vi "灯值调整对话框.vi"() -> ()   [LabVIEW 2016, in "斯坦道CODcr.lvlib"]
uses:
  <vilib>/Plasmionique/MB Master/MB_Master/MB_Master.lvclass
panel:
  out "工作状态:":string
  in  "纯水填充":bool
  out "660 阻值":u16 caption="660 阻值："
  out "520 阻值":u16 caption="520 阻值："
  out "365 阻值":u16 caption="365 阻值："
  in  "停止":bool
  in  "校准":bool
  out "校准状态":u16(ring) caption="调灯状态：" items=["空闲", "校准中"]
  out "当前阻值":u16 caption="当前阻值："
  out "当前光强":u16 caption="当前光强："
  in  "目标光强":u16=3300 caption="目标光强："
  in  "灯类型":enum32{"365", "520", "660"}(radio)=enum."660" caption="灯类型："
  # "365：海水氨氮\n520：海水氨氮、氨氮总磷（氨氮光源）\n660：总磷、氨氮"
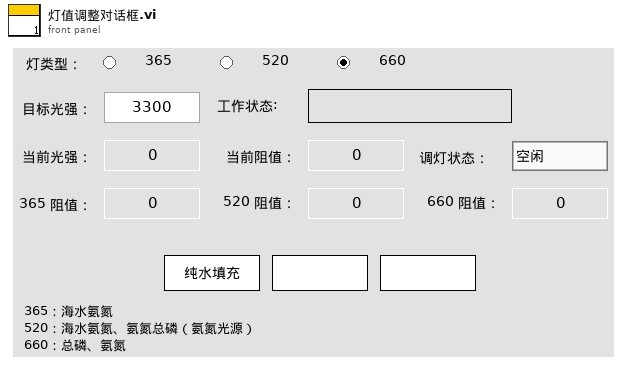
[diagram p1: front panel]
types:
  T1 = enum8{"Enabled", "Disabled", "Disabled and Grayed Out"}
  T2 = cluster{"系统时间":timestamp, "工作状态":u16, "测量模式":enum16{"待机", "连续模式", "周期模式", "定点模式", "受控模式", "手动模式"}, "告警代码":u16, "故障代码":u16, "日志代码":u16, "软件版本":u16, "F0":sgl, "F1":sgl, "F2":sgl, "F3":sgl, "T":sgl, "H":sgl, "id":u16, "flowid":u16, "量程":u16, "总磷控温温度1":sgl, "营养盐控温温度2":sgl, "ADC":sgl}
  T3 = cluster{"360 阻值":u16, "520 阻值":u16, "660 阻值":u16}
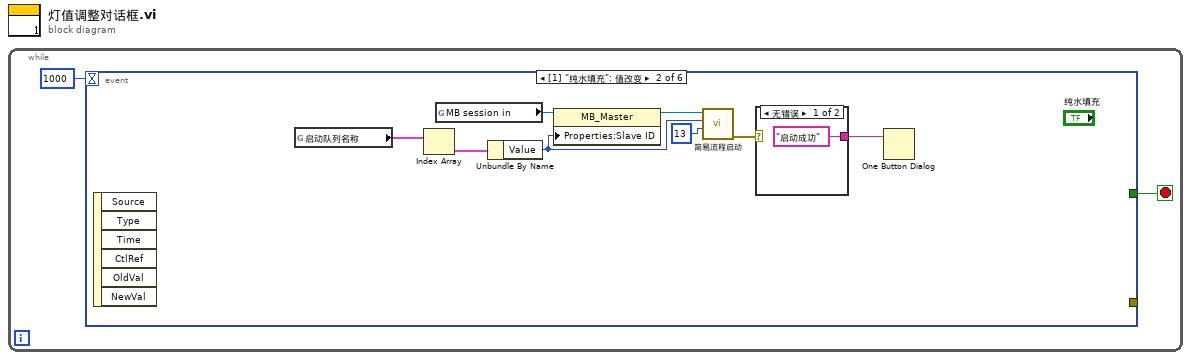
[diagram p0: block diagram]
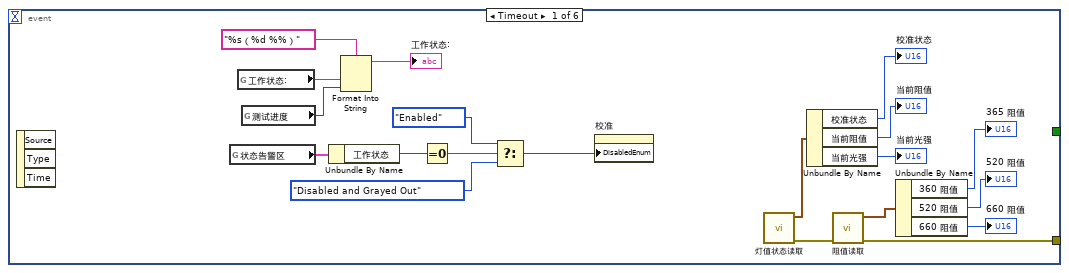
[diagram p2: hidden frame]
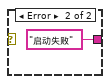
[diagram p3: hidden frame]
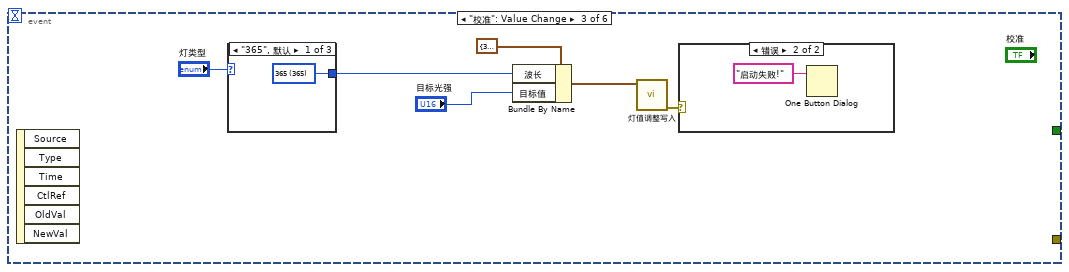
[diagram p4: hidden frame]
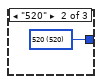
[diagram p6: hidden frame]
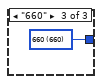
[diagram p7: hidden frame]
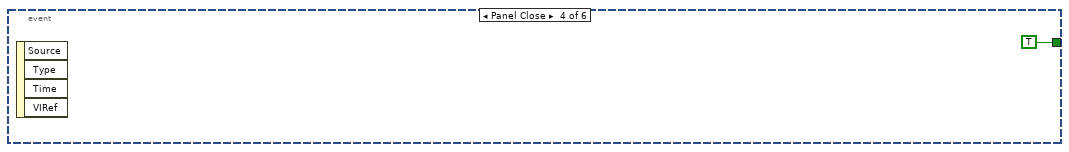
[diagram p8: hidden frame]
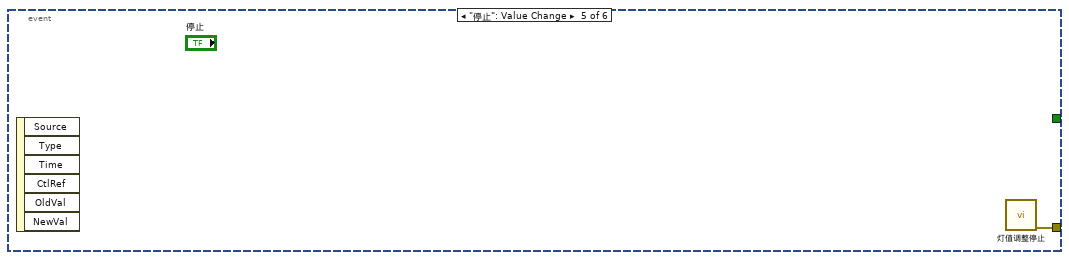
[diagram p9: hidden frame]
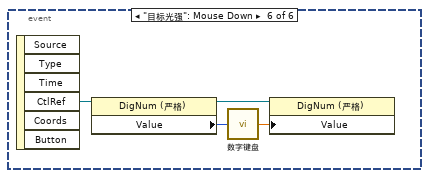
[diagram p10: hidden frame]
diagram:
  n1 = while {
    stop <- w2 stop-if-true
    n2 = event shown="[1] \"纯水填充\": 值改变" {
      selector: _ -> [_ _ _ _ _ _]
      dyn-events: _ -> [_ _ _ _ _ _]
      timeout: 1000 -> [_ _ _ _ _ _]
      tunnel: [_ _ _ TRUE _ _] -> w2
      tunnel: [w13 _ _ _ w44 _] -> _
      event Timeout {
        n3 = event-data() -> ()  [unwired: 1 in, 3 out]
        n4 = global read "VAR总磷总氮全局变量.vi" "状态告警区"() -> (w12:T2)
        n5 = global read "VAR总磷总氮全局变量.vi" "工作状态:"() -> (w5:string)
        n6 = global read "VAR总磷总氮全局变量.vi" "测试进度"() -> (w4:u8)
        n7 = Unbundle By Name(w12) -> ("工作状态"=w11:u16)
        n8 = Format Into String(format string="%s（%d %%）" ("格式字符串"), w5, w4) -> (resulting string=→"工作状态:":string)  [unwired: 2 in, 1 out]
        n9 = Equal To 0?(x=w11) -> (x = 0?=w10:bool)
        n10 = Select(t=T1."Enabled" ("禁用"), s=w10, f=T1."Disabled and Grayed Out") -> (s? t:f=w8:T1)
        n11 = property on="校准" class="Bool"("DisabledEnum"=w8) -> ()  [unwired: 2 in, 2 out]
        n12 = call "灯值状态读取.vi"() -> ("error out"=w22:errorcluster, "状态值"=w21:cluster{"校准状态":u16, "当前阻值":u16, "当前光强":u16})  [unwired: 10 in]
        n13 = Unbundle By Name(w21) -> ("校准状态"=→"校准状态":u16, "当前阻值"=→"当前阻值":u16, "当前光强"=→"当前光强":u16)
        n14 = call "阻值读取.vi"("error in (no error)"=w22) -> ("error out"=w13:errorcluster, "状态值"=w17:T3)  [unwired: 9 in]
        n15 = Unbundle By Name(w17) -> ("360 阻值"=→"365 阻值":u16, "520 阻值"=→"520 阻值":u16, "660 阻值"=→"660 阻值":u16)
      }
      event "纯水填充": Value Change {
        n16 = event-data() -> ()  [unwired: 1 in, 6 out]
        n17 = global read "model config var.vi" "启动队列名称"() -> (w25:cluster{"String":string, "Value":u16}[])
        n18 = Index Array(array=w25) -> (element=w24:cluster{"String":string, "Value":u16})  [unwired: 1 in]
        n19 = global read "VAR总磷总氮全局变量.vi" "MB session in"() -> (w28:refnum<class "MB_Master.lvclass">)
        n20 = Unbundle By Name(w24) -> ("Value"=w23:u16)
        n21 = property class="MB_Master"(reference=w28, "Properties:Slave ID"=w23) -> (reference out=w27:refnum<class "MB_Master.lvclass">)  [unwired: 1 in, 1 out]
        n22 = call "简易流程启动.vi"("简易流程"=13, "参数Id"=w23, "MB session in"=w27) -> ("error out"=w30:errorcluster)  [unwired: 7 in, 1 out]
        n23 = case shown="无错误" w30 {
          tunnel: ["启动成功" "启动失败"] -> w29
          frame No Error {
          }
          frame Error {
          }
        }
        n24 = One Button Dialog(message=w29) -> ()  [unwired: 1 in, 1 out]
      }
      event "校准": Value Change {
        n25 = event-data() -> ()  [unwired: 1 in, 6 out]
        n26 = case shown="\"365\", 默认" "灯类型" {
          tunnel: [w40 w41 w42] -> w33
          frame "365", Default {
            w40 = u16 365 items=["365"=365, "520"=520, "660"=660] ("波长")
          }
          frame "520" {
            w41 = u16 520 items=["365"=365, "520"=520, "660"=660] ("波长")
          }
          frame "660" {
            w42 = u16 660 items=["365"=365, "520"=520, "660"=660] ("波长")
          }
        }
        n27 = Bundle By Name(cluster=cluster{"波长":u16, "ADC":u16, "目标值":u16} {"波长"=365, "ADC"=0, "目标值"=0} ("写入值"), "波长"=w33, "目标值"="目标光强") -> (w35:cluster{"波长":u16, "ADC":u16, "目标值":u16})
        n28 = call "灯值调整写入.vi"("写入值"=w35) -> ("error out"=w36:errorcluster)  [unwired: 10 in]
        n29 = case shown="错误" w36 {
          frame No Error {
          }
          frame Error {
            n30 = One Button Dialog(message="启动失败!" ("消息")) -> ()  [unwired: 1 in, 1 out]
          }
        }
      }
      event Panel Close {
        n31 = event-data() -> ()  [unwired: 1 in, 4 out]
      }
      event "停止": Value Change {
        n32 = event-data() -> ()  [unwired: 1 in, 6 out]
        n33 = call "灯值调整停止.vi"() -> ("error out"=w44:errorcluster)  [unwired: 11 in]
      }
      event "目标光强": Mouse Down {
        n34 = event-data() -> ("CtlRef"=w48:refnum<vi>)  [unwired: 1 in, 5 out]
        n35 = property class="DigNum (严格)"(reference=w48) -> (reference out=w45:refnum<vi>, "Value"=w47:u16)  [unwired: 1 in, 1 out]
        n36 = call "数字键盘.vi"("OldNumber"=w47) -> ("NewNumber"=w46:dbl)
        n37 = property class="DigNum (严格)"(reference=w45, "Value"=w46) -> ()  [unwired: 1 in, 2 out]
      }
    }
  }
